vi "GCode_BasicVI.vi"(6 "Boolean in":bool, 9 "Array od string":string[](array[string]), 10 "Numeric control 2":i32, 11 "Numeric control":dbl) -> (0 "Waveform Chart":dbl(graph), 2 "Numeric indicator 2":i32, 3 "Numeric indicator":dbl)   [LabVIEW 2014]
panel:
  out "Boolean out":bool
  # "Inputs"
  # "Outputs"
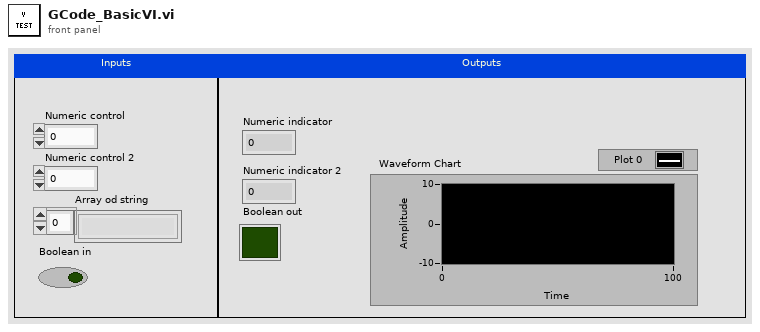
[diagram p1: front panel]
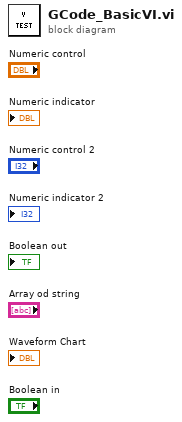
[diagram p0: block diagram]
diagram:
